vi "rgb to grayscale w IMAQ functions.vi"(7 "Convert Depth?":bool, 8 "error in (no error)":errorcluster, 10 "Processing Params":T1, 11 "Image In":T2) -> (0 "error out":errorcluster, 2 "Depth Values":dbl[][](array[numeric]), 3 "Image Out":T2, 4 "Elapsed Time (ms)":u32)   [LabVIEW 2018]
uses:
  <vilib>/vision/Image Controls.llb/IMAQ Image.ctl
  Processing Params STYP.ctl
  Pixel Data STYP.ctl
  Coordinate STYP.ctl
  Floating Pixel Data STYP.ctl
  <vilib>/vision/NI_Vision_Development_Module.lvlib
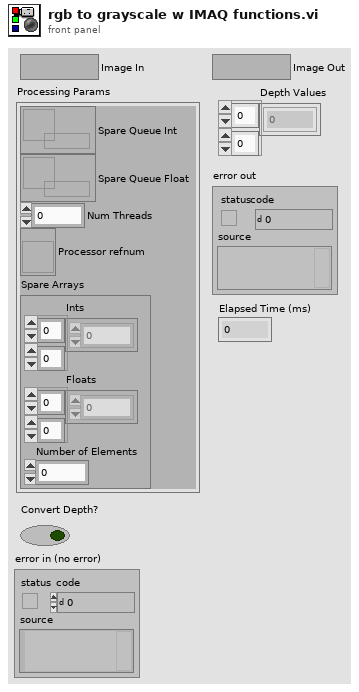
[diagram p1: front panel]
types:
  T1 = typedef "Processing Params STYP.ctl" = cluster{"Spare Queue Int":refnum<queue>, "Spare Queue Float":refnum<queue>, "Num Threads":i32, "Processor refnum":refnum<vi>, "Spare Arrays":cluster{"Ints":u8[][], "Floats":dbl[][], "Number of Elements":i32}}
  T2 = typedef "IMAQ Image.ctl" = refnum<image>
  T3 = typedef "Image Type" = u32
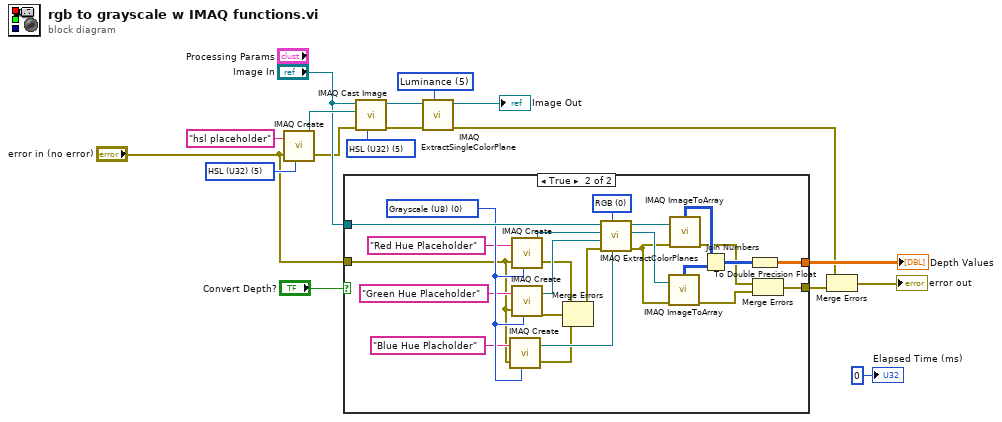
[diagram p0: block diagram]
diagram:
  w11 = T3 5 items=["Grayscale (U8)", "Grayscale (I16)", "Grayscale (SGL)", "Complex (CSG)", "RGB (U32)", "HSL (U32)", "RGB (U64)", "Grayscale (U16)"] ("Image Type")
  w15 = T3 5 items=["Grayscale (U8)", "Grayscale (I16)", "Grayscale (SGL)", "Complex (CSG)", "RGB (U32)", "HSL (U32)", "RGB (U64)", "Grayscale (U16)"] ("Image Type")
  w17 = 5 items=["Red", "Green", "Blue", "Hue", "Saturation", "Luminance", "Value", "Intensity"] ("Color Plane")
  n1 = call "IMAQ Create"("Image Name"="hsl placeholder", "Image Type"=w11, "error in (no error)"="error in (no error)") -> ("New Image"=w13:T2, "error out"=w7:errorcluster)  [unwired: 2 in]
  n2 = case shown="True" "Convert Depth?" {
    tunnel: "Image In" -> [_ w41]
    tunnel: [_ w27] -> w9
    tunnel: "error in (no error)" -> [_ w26]
    tunnel: [_ w18] -> w4
    frame False {
    }
    frame True {
      w31 = u16 0 items=["RGB", "HSL", "HSV", "HSI"] ("Color Mode")
      w37 = T3 0 items=["Grayscale (U8)", "Grayscale (I16)", "Grayscale (SGL)", "Complex (CSG)", "RGB (U32)", "HSL (U32)", "RGB (U64)", "Grayscale (U16)"] ("Image Type")
      n3 = call "IMAQ Create"("Image Name"="Blue Hue Placholder", "Image Type"=w37, "error in (no error)"=w26) -> ("New Image"=w38:T2, "error out"=w23:errorcluster)  [unwired: 2 in]
      n4 = call "IMAQ Create"("Image Name"="Red Hue Placeholder", "Image Type"=w37, "error in (no error)"=w26) -> ("New Image"=w40:T2, "error out"=w24:errorcluster)  [unwired: 2 in]
      n5 = call "IMAQ Create"("Image Name"="Green Hue Placeholder", "Image Type"=w37, "error in (no error)"=w26) -> ("New Image"=w39:T2, "error out"=w25:errorcluster)  [unwired: 2 in]
      n6 = Merge Errors(w24, w25, w23) -> (w22:errorcluster)
      n7 = call "IMAQ ExtractColorPlanes"("Blue or Luma or Val or Inten Plane"=w38, "Color Mode"=w31, "error in (no error)"=w22, "Green or Sat Plane"=w39, "Red or Hue Plane"=w40, "Image Src"=w41) -> ("error out"=w21:errorcluster, "Green or Sat Plane out"=w32:T2, "Red or Hue Plane out"=w33:T2)  [unwired: 2 in, 1 out]
      n8 = call "IMAQ ImageToArray"("error in (no error)"=w21, "Image"=w32) -> ("error out"=w19:errorcluster, "Image Pixels (U8)"=w29:u8[][])  [unwired: 2 in, 3 out]
      n9 = call "IMAQ ImageToArray"("error in (no error)"=w21, "Image"=w33) -> ("error out"=w20:errorcluster, "Image Pixels (U8)"=w30:u8[][])  [unwired: 2 in, 3 out]
      n10 = Join Numbers(hi=w30, lo=w29) -> ((hi.lo)=w28:u16[][])
      n11 = To Double Precision Float(number=w28) -> (double precision float=w27:dbl[][])
      n12 = Merge Errors(w20, w19) -> (w18:errorcluster)
    }
  }
  "Depth Values" <- w9
  n13 = call "IMAQ Cast Image"("Image Type"=w15, "error in (no error)"=w7, "Image Dst"=w13, "Image Src"="Image In") -> ("error out"=w6:errorcluster, "Image Dst Out"=w14:T2)  [unwired: 6 in]
  n14 = call "IMAQ ExtractSingleColorPlane"("Color Plane"=w17, "error in (no error)"=w6, "Image Src"=w14) -> ("error out"=w3:errorcluster, "Image Dst Out"=→"Image Out":T2)  [unwired: 7 in]
  n15 = Merge Errors(w3, w4) -> (→"error out":errorcluster)
  "Elapsed Time (ms)" <- u32 0 ("Elapsed Time (ms)")
